vi "AddContained.vi"(8 "error in (no error)":errorcluster, 9 "Item to contain":refnum<class "ILabVIEWItem.lvclass">, 11 "CLabVIEWContainer in":refnum<class "CLabVIEWContainer.lvclass">) -> (0 "error out":errorcluster, 1 "Relationship type":T1, 3 "CLabVIEWContainer out":refnum<class "CLabVIEWContainer.lvclass">)   [LabVIEW 2020, in "LabVIEWContainers.lvlib" / "CLabVIEWContainer.lvclass"]
uses:
  CLabVIEWContainer.lvclass
  obj/Addons/LabVIEWObjectInterfaces.lvlibp/LabVIEWObjectInterfaces/ILabVIEWItem/ILabVIEWItem.lvclass
  obj/Addons/LabVIEWObjectInterfaces.lvlibp/LabVIEWObjectInterfaces/ILabVIEWItem/RelationshipType.ctl
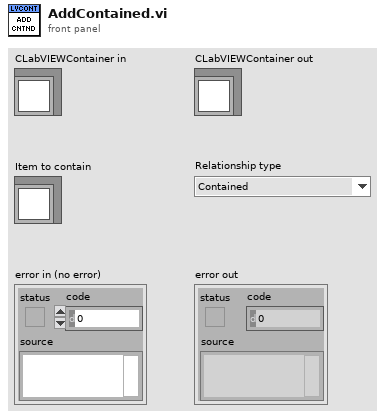
[diagram p1: front panel]
types:
  T1 = typedef "LabVIEWObjectInterfaces.lvlibp/ILabVIEWItem.lvclass/RelationshipType.ctl" = enum16{"Contained", "Dependency", "Parent", "Same item", "Related", "None"}
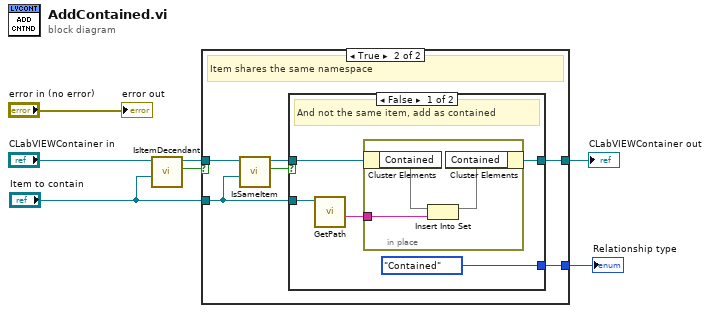
[diagram p0: block diagram]
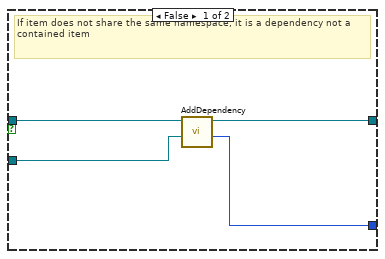
[diagram p2: hidden frame]
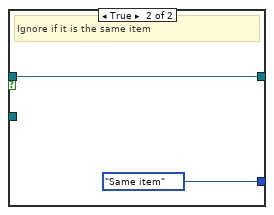
[diagram p3: hidden frame]
diagram:
  n1 = call-dynamic "IsItemDecendant.vi"("Item to compare"="Item to contain", "CLabVIEWItem in"="CLabVIEWContainer in") -> ("Is a decendant?"=w2:bool, "CLabVIEWItem out"=w4:refnum<class "CLabVIEWContainer.lvclass">)  [unwired: 7 in, 1 out]
  n2 = case shown="True" w2 {
    tunnel: [w10 w17] -> w7
    tunnel: w4 -> [w11 w16]
    tunnel: "Item to contain" -> [w9 w14]
    tunnel: [w8 w12] -> w1
    frame False {
      # "If item does not share the same namespace, it is a dependency not a contained item"
      n3 = call-dynamic "AddDependency.vi"("Item to depend on"=w9, "CLabVIEWItem in"=w11) -> ("Relationship type"=w8:T1, "CLabVIEWItem out"=w10:refnum<class "CLabVIEWContainer.lvclass">)  [unwired: 7 in, 1 out]
    }
    frame True {
      # "Item shares the same namespace"
      n4 = call-dynamic "IsSameItem.vi"("Compare to item"=w14, "CLabVIEWItem in"=w16) -> ("Is same?"=w13:bool, "CLabVIEWItem out"=w15:refnum<class "CLabVIEWContainer.lvclass">)  [unwired: 7 in, 1 out]
      n5 = case shown="False" w13 {
        tunnel: [w22 w27] -> w17
        tunnel: w15 -> [w20 w27]
        tunnel: w14 -> [w19 _]
        tunnel: [RelationshipType."Contained" ("Relationship type") RelationshipType."Same item" ("Relationship type")] -> w12
        frame False {
          # "And not the same item, add as contained"
          n6 = call-dynamic "GetPath.vi"("ILabVIEWItem in"=w19) -> ("Path"=w21:string)  [unwired: 8 in, 2 out]
          n7 = in-place {
            in-place-border: w21 -> [w23]
            n8 = in-place-cluster #1(w20) -> ("Contained"=w24:set{string})
            n9 = Insert Into Set(10:w23, 11:w24) -> (3:w25:set{string})  [unwired: 1 out]
            n10 = in-place-cluster #1("Contained"=w25) -> (w22:refnum<class "CLabVIEWContainer.lvclass">)
          }
        }
        frame True {
          # "Ignore if it is the same item"
        }
      }
    }
  }
  "CLabVIEWContainer out" <- w7
  "Relationship type" <- w1
  "error out" <- "error in (no error)"
